vi "N9310A Sweep LF Out.vi"() -> ()   [LabVIEW 2018]
uses:
  <instrlib>/Agilent N9310/Agilent N9310.lvlib
panel:
  in  "VISA resource name of Agilent N9310A":refnum<visa-resource-name>
  in  "Wait between steps (s)":dbl=1.0 format="%#_6p"
  out "Current step":dbl format="%^#_6e"
  out "Current frequency":dbl format="%#_6p"
  in  "Steps":dbl=16.0 format="%^#_6e"
  in  "Amplitude (V)":dbl=0.5 format="%#_6p"
  in  "End frequency (Hz)":dbl=1200.0 format="%#_6p"
  in  "Start frequency (Hz)":dbl=800.0 format="%#_6p"
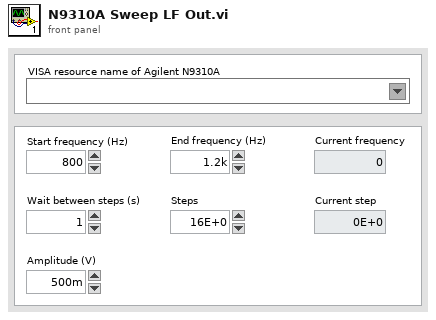
[diagram p1: front panel]
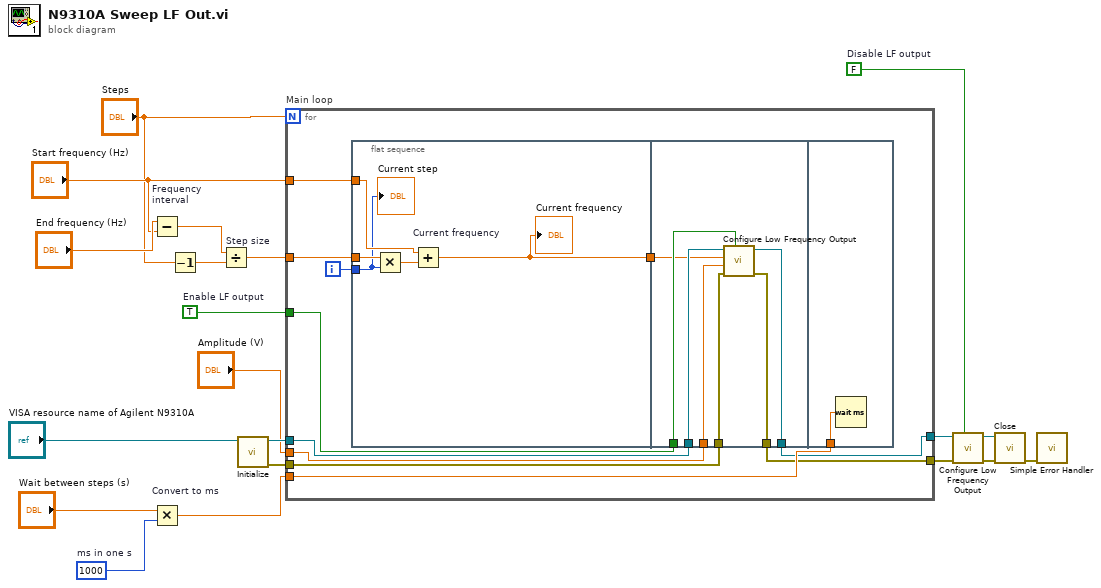
[diagram p0: block diagram]
diagram:
  w1 = FALSE  # Disable LF output
  w8 = TRUE  # Enable LF output
  w14 = 1000  # ms in one s
  n1 = Subtract "Frequency\ninterval"(x="End frequency (Hz)", y="Start frequency (Hz)") -> (x-y=w19:dbl)
  n2 = Multiply "Convert to ms"(x="Wait between steps (s)", y=w14) -> (x*y=w16:dbl)
  n3 = Decrement(x="Steps") -> (x-1=w12:dbl)
  n4 = Divide "Step size"(x=w19, y=w12) -> (x/y=w18:dbl)
  n5 = call <instrlib>:"Initialize.vi"("VISA resource name"="VISA resource name of Agilent N9310A") -> ("error out"=w9:errorcluster, "VISA resource name out"=w10:refnum<visa-resource-name>)  [unwired: 9 in]
  n6 = for "Main loop" {
    N: "Steps" -> [_]
    tunnel: w18 -> [w31]
    tunnel: "Start frequency (Hz)" -> [w30]
    tunnel: w16 -> [w29]
    tunnel: w10 -> [w28]
    tunnel: w9 -> [w27]
    tunnel: w8 -> [w26]
    tunnel: "Amplitude (V)" -> [w24]
    tunnel: [w23] -> w5
    tunnel: [w22] -> w4
    i -> [w21]
    n7 = flat-sequence {
      tunnel: w21 -> [w32]
      tunnel: w31 -> [w35]
      tunnel: w30 -> [w34]
      tunnel: [w33] -> w25
      tunnel: w28 -> [w43]
      tunnel: w27 -> [w42]
      tunnel: w26 -> [w41]
      tunnel: w25 -> [w40]
      tunnel: w24 -> [w39]
      tunnel: [w38] -> w23
      tunnel: [w37] -> w22
      tunnel: w29 -> [w44]
      frame #0 {
        n8 = Multiply(x=w35, y=w32) -> (x*y=w36:dbl)
        n9 = Add "Current frequency"(x=w34, y=w36) -> (x+y=w33:dbl)
        "Current frequency" <- w33
        "Current step" <- w32
      }
      frame #1 {
        n10 = call <instrlib>:"Configure Low Frequency Output.vi"("Enable LF Output (F:Disable)"=w41, "error in (no error)"=w42, "Amplitude (0.5 V)"=w39, "Frequency (1.0 kHz)"=w40, "VISA resource name"=w43) -> ("error out"=w37:errorcluster, "VISA resource name out"=w38:refnum<visa-resource-name>)  [unwired: 5 in]
      }
      frame #2 {
        n11 = Wait (ms)(milliseconds to wait=w44) -> ()  [unwired: 1 out]
      }
    }
  }
  n12 = call <instrlib>:"Configure Low Frequency Output.vi"("Enable LF Output (F:Disable)"=w1, "error in (no error)"=w4, "VISA resource name"=w5) -> ("error out"=w2:errorcluster, "VISA resource name out"=w3:refnum<visa-resource-name>)  [unwired: 7 in]
  n13 = call <instrlib>:"Close.vi"("error in (no error)"=w2, "VISA resource name"=w3) -> ("error out"=w6:errorcluster)  [unwired: 9 in]
  n14 = call <vilib>:"Simple Error Handler.vi"("error in (no error)"=w6) -> ()  [unwired: 4 in, 5 out]
